vi "extractElementName.vi"(8 "error in (no error)":errorcluster, 11 "Topic in":refnum<class "Topic.lvclass">) -> (0 "error out":errorcluster, 2 "elementName":string, 3 "Topic out":refnum<class "Topic.lvclass">)   [LabVIEW 2013, in "Topic.lvclass"]
uses:
  Topic.lvclass
  Topic.lvclass/Topic.ctl
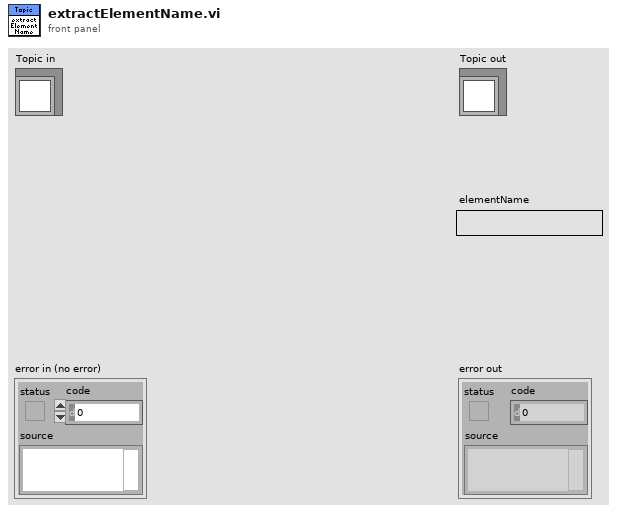
[diagram p1: front panel]
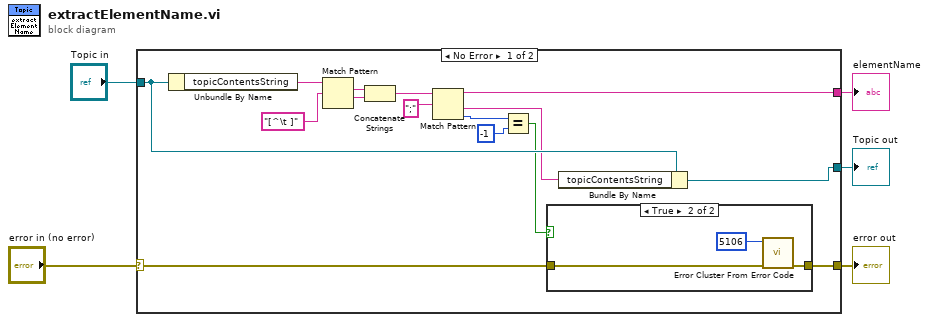
[diagram p0: block diagram]
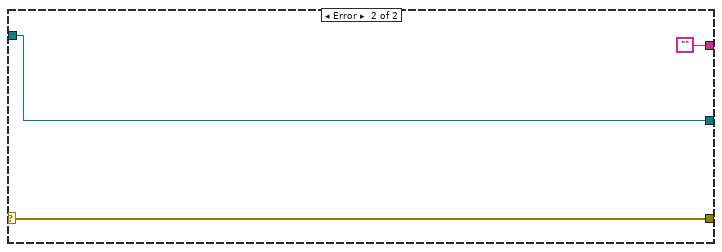
[diagram p3: hidden frame]
diagram:
  n1 = case shown="No Error" "error in (no error)" {
    selector: "error in (no error)" -> [w9 w27]
    tunnel: [w7 w27] -> w4
    tunnel: [w11 w26] -> w2
    tunnel: "Topic in" -> [w12 w26]
    tunnel: [w10 ""] -> w1
    frame No Error {
      n2 = Unbundle By Name(w12) -> ("topicContentsString"=w13:string)
      n3 = Match Pattern(string=w13, regular expression="[^\t ]") -> (match substring=w16:string, after substring=w15:string)  [unwired: 1 in, 2 out]
      n4 = Concatenate Strings(w16, w15) -> (w14:string)
      n5 = Match Pattern(string=w14, regular expression=";") -> (before substring=w10:string, after substring=w6:string, offset past match=w19:i32)  [unwired: 1 in, 1 out]
      n6 = Equal?(x=w19, y=-1) -> (x = y?=w8:bool)
      n7 = case shown="True" w8 {
        tunnel: w9 -> [w21 w24]
        tunnel: [w21 w23] -> w7
        frame False {
        }
        frame True {
          n8 = call <vilib>:"Error Cluster From Error Code.vi"("error in (no error)"=w24, "error code (0)"=5106) -> ("error out"=w23:errorcluster)  [unwired: 7 in]
        }
      }
      n9 = Bundle By Name(cluster=w12, "topicContentsString"=w6) -> (w11:refnum<class "Topic.lvclass">)
    }
    frame Error {
    }
  }
  "error out" <- w4
  "Topic out" <- w2
  "elementName" <- w1
